vi "Command Sequencer.vi"(9 "Iterations":dbl format="%#_13g", 11 "Commands":cluster{"Time (s)":dbl, T1, bool}[](array[cluster])) -> ()   [LabVIEW 2019]
uses:
  Bordeaux/bordeaux-pathinator/Bordeaux/Command Stuff/Single Cmd Info.ctl
  <vilib>/picture/picture.llb/imagedata.ctl
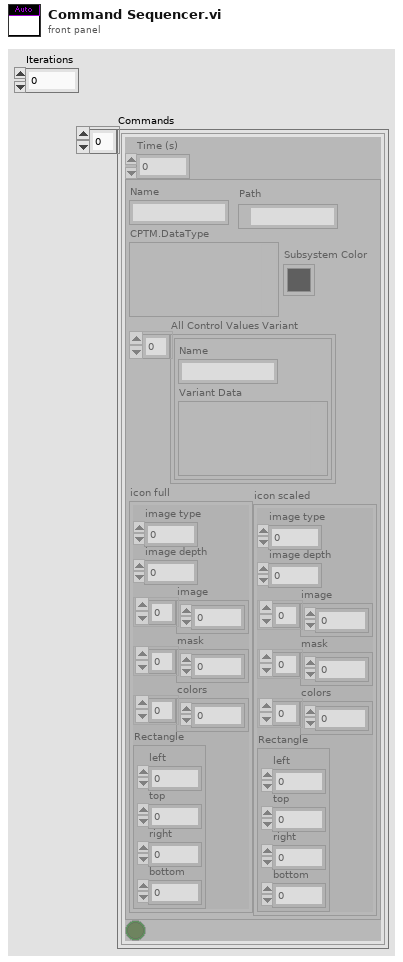
[diagram p1: front panel]
types:
  T1 = typedef "Single Cmd Info.ctl" = cluster{"Name":string, "CPTM.DataType":variant, "All Control Values Variant":cluster{"Name":string, "Variant Data":variant}[], "icon full":T2, "icon scaled":T2, "Path":path, "Subsystem Color":u32}
  T2 = typedef "imagedata.ctl" = cluster{"image type":i32, "image depth":i32, "image":u8[], "mask":u8[], "colors":u32[], "Rectangle":cluster{"left":i16, "top":i16, "right":i16, "bottom":i16}}
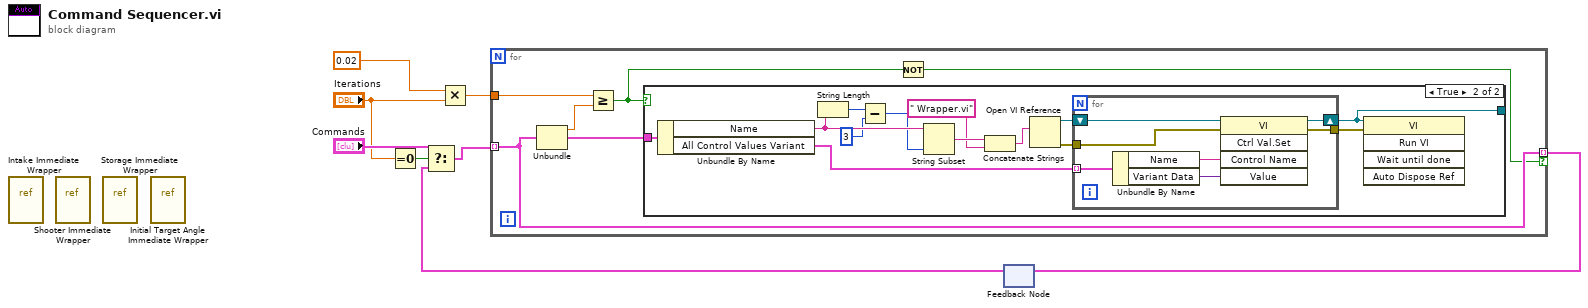
[diagram p0: block diagram]
diagram:
  n1 = vi-ref "Intake Immediate Wrapper.vi"() -> ()  [unwired: 1 out]
  n2 = vi-ref "Shooter Immediate Wrapper.vi"() -> ()  [unwired: 1 out]
  n3 = vi-ref "Storage Immediate Wrapper.vi"() -> ()  [unwired: 1 out]
  n4 = vi-ref "Initial Target Angle Immediate Wrapper.vi"() -> ()  [unwired: 1 out]
  n5 = Equal To 0?(x="Iterations") -> (x = 0?=w4:bool)
  n6 = Multiply(x=0.02, y="Iterations") -> (x*y=w7:dbl)
  n7 = feedback #1() -> (w1:cluster{"Time (s)":dbl, T1, bool}[])  [unwired: 1 in]
  n8 = Select(t="Commands", s=w4, f=w1) -> (s? t:f=w3:cluster{"Time (s)":dbl, T1, bool}[])
  n9 = for {
    tunnel: w7 -> [w14]
    tunnel: w3 -> [w10] mode=indexing
    tunnel: [w10] -> w2 mode=indexing if=w9
    n10 = Unbundle(w10) -> ("Time (s)"=w12:dbl, w13:T1)  [unwired: 1 out]
    n11 = Greater Or Equal?(x=w14, y=w12) -> (x >= y?=w11:bool)
    n12 = case shown="True" w11 {
      tunnel: w13 -> [_ w23]
      tunnel: [_ w15] -> _
      frame False {
      }
      frame True {
        n13 = Unbundle By Name(w23) -> ("Name"=w22:string, "All Control Values Variant"=w26:cluster{"Name":string, "Variant Data":variant}[])
        n14 = String Length(string=w22) -> (length=w21:i32)
        n15 = Subtract(x=w21, y=3) -> (x-y=w19:i32)
        n16 = String Subset(string=w22, length (rest)=w19) -> (substring=w18:string)  [unwired: 1 in]
        n17 = Concatenate Strings(w18, " Wrapper.vi" ("string")) -> (w16:string)
        n18 = Open VI Reference(vi path=w16) -> (vi reference=w27:refnum<vi>, error out=w25:errorcluster)  [unwired: 5 in]
        n19 = for {
          shift-right: [w33] -> w15
          shift-left: w27 -> [w34]
          tunnel: w26 -> [w29] mode=indexing
          tunnel: w25 -> [w31]
          tunnel: [w30] -> w24
          n20 = Unbundle By Name(w29) -> ("Name"=w28:string, "Variant Data"=w32:variant)
          n21 = invoke class="VI" method="Ctrl Val.Set"(reference=w34, error in=w31, "Control Name"=w28, "Value"=w32) -> (reference out=w33:refnum<vi>, error out=w30:errorcluster)  [unwired: 1 in, 3 out]
        }
        n22 = invoke class="VI" method="Run VI"(reference=w15, error in=w24) -> ()  [unwired: 3 in, 5 out]
      }
    }
    n23 = Not(x=w11) -> (.not. x?=w9:bool)
  }
  n24 = feedback-in #1(w2) -> ()
